vi "Send Stop Message.vi"(8 "error in (no error)":errorcluster, 11 "Execute":refnum<class "Execute.lvclass">) -> (0 "error out":errorcluster, 3 "Execute":refnum<class "Execute.lvclass">)   [LabVIEW 2018, in "QMH_Class.lvlib" / "TestManager.lvlib" / "Stop Message.lvclass"]
uses:
  Stop Message.lvclass
  Execute_class/Execute.lvclass
  E:/0 File/GITSync/DynoToolPlus/0 LabviewCode/0 Support/Message Queue_Class/Class/Message_class/InterfaceMessage/Interface Message.lvclass
  Execute_class/Execute.lvclass/Execute.ctl
  InterfaceMessage/Interface Message.lvclass
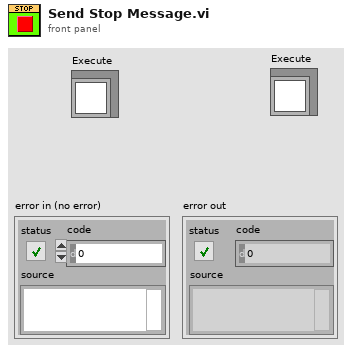
[diagram p1: front panel]
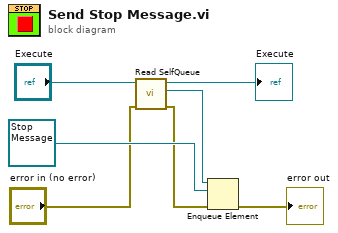
[diagram p0: block diagram]
diagram:
  n1 = call "Read SelfQueue.vi"("error in (no error)"="error in (no error)", "Execute"="Execute") -> ("error out"=w1:errorcluster, "SelfQueue"=w4:refnum<queue>, "Execute"=→"Execute":refnum<class "Execute.lvclass">)  [unwired: 7 in]
  n2 = Enqueue Element(queue=w4, element=refnum<class "Stop Message.lvclass"> refnum ("Actor.lvlib:Stop Message.lvclass"), error in (no error)=w1) -> (error out=→"error out":errorcluster)  [unwired: 1 in, 2 out]
